vi "ESA-C Objective Transform.vi"(2 "Axis":i32=1 min=1 max=3 step=1, 3 "Is Voltage?":bool, 4 "Input Value":dbl) -> (1 "Output Value":dbl)   [LabVIEW 2010]
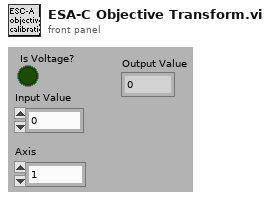
[diagram p1: front panel]
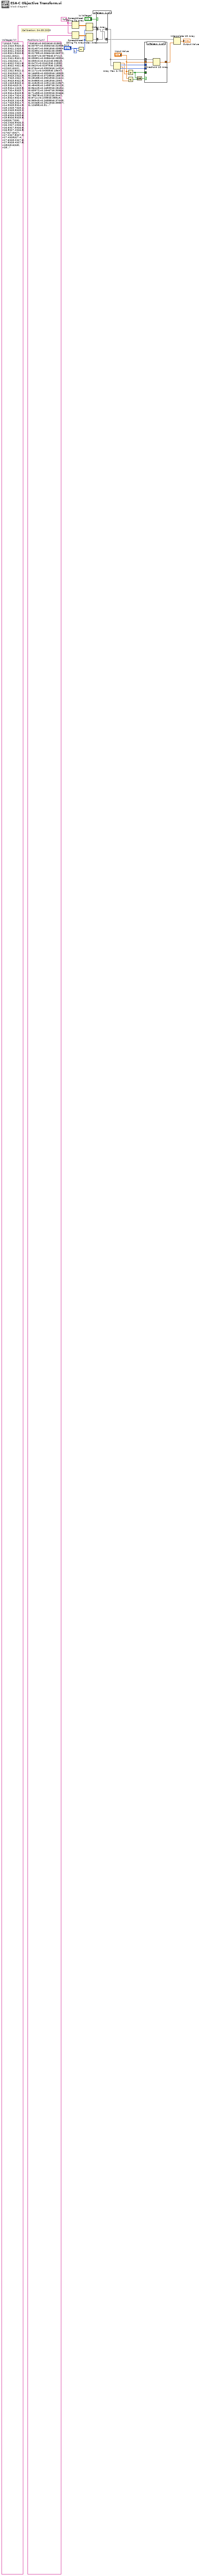
[diagram p0: block diagram]
diagram:
  w2 = "%f" ("Format-String")
  w4 = "0\t0\t0\n0.00206\t0.01582\t0.00797\n0.00364\t0.02598\t0.01407\n0.00618\t0.03864\t0.02391\n0.00461\t0.0389\t0.01785\n0.00664\t0.06372\t0.0257\n0.00796\t0.07414\t0.03081\n0.00864\t0.08594\t0.03344\n0.0122\t0.09613\t0.0472\n0.01613\t0.11592\t0.0624\n0.01975\t0.12826\t0.07644\n0.03026\t0.14314\t0.1171\n0.04305\t0.15647\t0.16659\n0.05309\t0.18503\t0.20543\n0.07285\t0.18573\t0.28188\n0.09015\t0.21641\t0.34883\n0.10815\t0.2394\t0.41849\n0.12511\t0.24567\t0.48409\n0.14587\t0.26123\t0.56443\n0.16533\t0.28494\t0.63972\n0.18467\t0.30966\t0.71458\n0.20333\t0.32666\t0.78678\n0.22512\t0.3447\t0.8711\n0.2495\t0.35813\t0.96543\n0.26998\t0.37045\t1.04468\n0.29125\t0.39557\t1.12698\n0.31199\t0.43186\t1.20721\n0.33041\t0.44995\t1.2785\n0.35642\t0.46128\t1.37913\n0.37679\t0.4852\t1.45795\n0.39894\t0.51012\t1.54367\n0.423\t0.53809\t1.63678\n0.44765\t0.55311\t1.73215\n0.47119\t0.5793\t1.82326\n0.49323\t0.60432\t1.90852\n0.515\t0.63131\t1.99277\n0.54235\t0.65174\t2.0986\n0.56544\t0.67444\t2.18794\n0.59052\t0.70035\t2.28499\n0.61768\t0.72617\t2.39006\n0.64687\t0.74807\t2.50303\n0.67071\t0.77736\t2.59525\n0.69695\t0.79842\t2.69682\n0.72326\t0.82413\t2.79861\n0.75249\t0.851\t2.91173\n0.77818\t0.86434\t3.01111\n0.80787\t0.89958\t3.12601\n0.83626\t0.92291\t3.23587\n0.86609\t0.9444\t3.35128\n0.89348\t0.97648\t3.45728\n0.92459\t1.01656\t3.57766\n0.95407\t1.03769\t3.69172\n0.98644\t1.06928\t3.81698\n1.0145\t1.08591\t3.92557\n1.05304\t1.12184\t4.07469\n1.08169\t1.16283\t4.18554\n1.11425\t1.17713\t4.31154\n1.14477\t1.23843\t4.42962\n1.17871\t1.2712\t4.56095\n1.21176\t1.26837\t4.68883\n1.24316\t1.2797\t4.81034\n1.27406\t1.35775\t4.92992\n1.306\t1.35966\t5.05349\n1.34587\t1.39661\t5.20777\n1.37659\t1.41265\t5.32665\n1.41003\t1.45457\t5.45604\n1.44185\t1.47975\t5.57914\n1.4793\t1.5145\t5.72406\n1.51209\t1.54856\t5.85095\n1.54619\t1.57829\t5.98287\n1.58446\t1.61345\t6.13097\n1.62127\t1.64402\t6.27342\n1.65394\t1.68094\t6.39983\n1.6971\t1.71433\t6.56684\n1.7329\t1.75848\t6.70537\n1.77332\t1.78004\t6.86175\n1.80796\t1.82347\t6.9958\n1.84327\t1.8469\t7.13243\n1.88063\t1.88883\t7.27699\n1.91665\t1.92539\t7.41636\n1.95809\t1.95381\t7.5767\n1.99357\t1.99138\t7.71401\n2.03643\t2.02811\t7.87986\n2.07282\t2.065\t8.02067\n2.11601\t2.10377\t8.18776\n2.15509\t2.14263\t8.33898\n2.19327\t2.17343\t8.48672\n2.23173\t2.20447\t8.63557\n2.27341\t2.23879\t8.79684\n2.31601\t2.27513\t8.96165\n2.35787\t2.31235\t9.12363\n2.39614\t2.3465\t9.27174\n2.44248\t2.40021\t9.45105\n2.4776\t2.44355\t9.58695\n2.52469\t2.44838\t9.76913\n2.56468\t2.51196\t9.92388\n2.60903\t2.54639\t10.0955\n2.65291\t2.5898\t10.2653\n2.69732\t2.63336\t10.43714\n2.73913\t2.65922\t10.59892\n2.78379\t2.70832\t10.77172\n2.82858\t2.74906\t10.94503\n2.86806\t2.77566\t11.0978\n2.91738\t2.8185\t11.28862\n2.96297\t2.8658\t11.46503\n3.00445\t2.90357\t11.62554\n3.05282\t2.95446\t11.81271\n3.09734\t2.98834\t11.98499\n3.14164\t3.02822\t12.1564\n3.18598\t3.06209\t12.32798\n3.2341\t3.1123\t12.51415\n3.27896\t3.14462\t12.68776\n3.32286\t3.18405\t12.8576\n3.37437\t3.23418\t13.05692\n3.41886\t3.27317\t13.22909\n3.4663\t3.32029\t13.41266\n3.51342\t3.34422\t13.59498\n3.55833\t3.39015\t13.76876\n3.61246\t3.42698\t13.97821\n3.6588\t3.47641\t14.15752\n3.70534\t3.51359\t14.33761\n3.75632\t3.57169\t14.53486\n3.80315\t3.59949\t14.71609\n3.85382\t3.64781\t14.91212\n3.89979\t3.69649\t15.09003\n3.94977\t3.73421\t15.28341\n4.00091\t3.77877\t15.4813\n4.04792\t3.82143\t15.6632\n4.09999\t3.87226\t15.86468\n4.14481\t3.918\t16.0381\n4.19552\t3.95085\t16.23433\n4.24804\t4.00483\t16.43755\n4.29611\t4.04561\t16.62355\n4.3445\t4.08787\t16.81079\n4.39609\t4.14791\t17.01041\n4.4472\t4.17144\t17.20818\n4.49829\t4.21375\t17.40587\n4.54788\t4.26894\t17.59774\n4.60011\t4.31296\t17.79985\n4.6533\t4.3514\t18.00569\n4.70481\t4.40255\t18.20499\n4.75815\t4.44984\t18.41138\n4.80998\t4.49487\t18.61196\n4.85901\t4.53422\t18.80166\n4.91528\t4.57675\t19.0194\n4.96618\t4.62801\t19.21633\n5.02209\t4.6768\t19.43268\n5.07231\t4.7086\t19.62702\n5.12469\t4.75743\t19.8297\n5.17561\t4.80586\t20.02672\n5.22927\t4.86141\t20.23436\n5.27506\t4.91224\t20.41152\n5.32744\t4.95287\t20.61423\n5.384\t4.99441\t20.83309\n5.43428\t5.03405\t21.02761\n5.48864\t5.0793\t21.23798\n5.54097\t5.13635\t21.44046\n5.59504\t5.17679\t21.6497\n5.64706\t5.2266\t21.85099\n5.70423\t5.263\t22.07218\n5.75231\t5.30995\t22.25823\n5.80554\t5.35144\t22.46421\n5.85792\t5.4046\t22.66688\n5.91238\t5.44471\t22.87761\n5.9677\t5.49265\t23.09165\n6.02253\t5.53708\t23.30384\n6.07348\t5.58112\t23.50097\n6.12782\t5.63989\t23.71125\n6.17763\t5.6757\t23.90398\n6.23196\t5.71507\t24.11421\n6.2856\t5.76459\t24.32178\n6.33948\t5.81711\t24.53024\n6.39054\t5.84114\t24.72783\n6.44988\t5.87321\t24.95743\n6.50485\t5.94542\t25.17015\n6.55614\t5.99001\t25.36861\n6.60972\t6.03117\t25.57592\n6.66579\t6.07023\t25.79287\n6.71452\t6.1316\t25.98144\n6.76881\t6.1573\t26.19152\n6.82217\t6.24148\t26.39801\n6.87766\t6.24631\t26.61272\n6.93251\t6.29414\t26.82493\n6.98672\t6.34088\t27.03473\n7.04211\t6.39186\t27.24903\n7.09161\t6.42876\t27.44056\n7.14462\t6.48125\t27.64568\n7.20275\t6.52643\t27.87062\n7.2513\t6.56734\t28.0585\n7.30852\t6.61388\t28.27988\n7.36287\t6.65737\t28.49019\n7.41237\t6.71161\t28.68175\n7.46672\t6.7582\t28.89205\n7.52048\t6.764\t29.10006\n7.57284\t6.8349\t29.30268\n7.62522\t6.87743\t29.50533\n7.67605\t6.92471\t29.70205\n7.73309\t6.979\t29.92274\n7.78587\t7.00484\t30.12696\n7.83692\t7.00877\t30.32451\n7.88874\t7.11708\t30.52503\n7.94425\t7.15008\t30.73983\n8.0003\t7.19203\t30.95672\n8.05026\t7.17301\t31.15001\n8.10258\t7.3525\t31.35245\n8.15648\t7.25315\t31.56101\n8.20663\t7.32632\t31.75506\n8.25782\t7.38747\t31.95315\n8.31409\t7.46022\t32.1709\n8.36985\t7.47799\t32.38664\n8.42199\t7.52294\t32.58842\n8.47558\t7.55001\t32.79578\n8.52455\t7.61783\t32.98525\n8.58088\t7.65449\t33.20322\n8.63041\t7.69981\t33.39486\n8.6828\t7.7452\t33.59759\n8.73825\t7.78797\t33.81217\n8.78556\t7.83191\t33.99523\n8.83822\t7.87419\t34.19896\n8.89339\t7.91015\t34.41248\n8.94467\t7.95395\t34.61087\n9.00029\t8.00004\t34.82609\n9.04789\t8.04302\t35.01028\n9.10104\t8.08233\t35.21594\n9.15413\t8.12348\t35.42139\n9.2035\t8.16484\t35.61243\n9.25364\t8.16852\t35.80641\n9.30931\t8.28485\t36.02185\n9.35645\t8.30373\t36.20425\n9.41107\t8.32962\t36.41559\n9.46247\t8.38694\t36.61447\n9.51232\t8.42657\t36.80736\n9.56033\t8.48788\t36.99315\n9.61139\t8.50867\t37.19072\n9.66139\t8.5305\t37.38418\n9.71153\t8.58622\t37.57821\n9.76035\t8.58666\t37.76709\n9.81322\t8.67561\t37.97169\n9.86271\t8.74104\t38.16319\n9.91232\t8.71631\t38.35513\n9.96116\t8.82303\t38.54412\n10.0396\t8.81323\t38.75433\n10.11293\t8.86917\t38.94097\n10.16317\t8.90354\t39.1314\n10.21362\t8.91815\t39.32582\n10.26417\t8.97055\t39.521\n10.31629\t9.0306\t39.7166\n10.36417\t9.09231\t39.91828\n10.4393\t9.09117\t40.10356\n10.51016\t9.13577\t40.30034\n10.56212\t9.19679\t40.48822\n10.6101\t9.23739\t40.66847\n10.65723\t9.27728\t40.86953\n10.70656\t9.31648\t41.05516\n10.75729\t9.32865\t41.23752\n10.80621\t9.38383\t41.4284\n10.85248\t9.42618\t41.62471\n10.90259\t9.44632\t41.814\n10.9494\t9.52148\t41.99304\n10.99657\t9.53135\t42.18693\n11.04455\t9.59795\t42.36807\n11.09076\t9.62348\t42.5506\n11.13748\t9.66961\t42.73625\n11.18797\t9.70076\t42.91506\n11.23827\t9.73559\t43.09583\n11.28985\t9.7884\t43.29121\n11.32964\t9.81555\t43.48582\n11.38187\t9.85709\t43.68541\n11.42597\t9.90824\t43.83939\n11.47253\t9.97563\t44.04148\n11.524\t9.99489\t44.21214\n11.57492\t10.02446\t44.3923\n11.62449\t10.06307\t44.59143\n11.67333\t10.10766\t44.7885\n11.71995\t10.15172\t44.98028\n11.76875\t10.18305\t45.16927\n11.81213\t10.22079\t45.34967\n11.86182\t10.25701\t45.53851\n11.90706\t10.29925\t45.70636\n11.95348\t10.34037\t45.89862\n11.9998\t10.38086\t46.07367\n12.05592\t10.41878\t46.2533\n12.09164\t10.45961\t46.43253\n12.13693\t10.49808\t46.64969\n12.18385\t10.51628\t46.78791\n12.22765\t10.57388\t46.96315\n12.2773\t10.61827\t47.14471\n12.32159\t10.65369\t47.31417\n12.36563\t10.701\t47.50632\n12.41129\t10.72273\t47.67768\n12.45403\t10.78257\t47.84809\n12.49792\t10.81064\t48.02478\n12.54281\t10.85043\t48.19016\n12.58755\t10.88123\t48.35996\n12.63056\t10.93561\t48.53366\n12.67788\t10.95375\t48.70681\n12.7214\t11.00172\t48.87324\n12.76449\t11.0412\t49.05632\n12.80979\t11.07308\t49.22472\n12.85226\t11.11637\t49.39145\n12.90002\t11.16052\t49.56675\n12.93855\t11.19604\t49.73109\n12.98328\t11.23555\t49.9159\n13.03221\t11.26792\t50.06498\n13.07624\t11.30576\t50.23803\n13.1182\t11.35628\t50.42737\n13.16017\t11.38331\t50.59777\n13.21028\t11.42008\t50.76012\n13.25055\t11.46065\t50.9225\n13.2949\t11.49544\t51.11642\n13.33123\t11.54413\t51.27223\n13.37735\t11.5857\t51.44383\n13.418\t11.62174\t51.58444\n13.46358\t11.6533\t51.7629\n13.51193\t11.70144\t51.92018\n13.54756\t11.73269\t52.09654\n13.59149\t11.76663\t52.28364\n13.63076\t11.80746\t52.42152\n13.67299\t11.8394\t52.59147\n13.73724\t11.88143\t52.74344\n13.79991\t11.92458\t52.90683\n13.83781\t11.95047\t53.07778\n13.88384\t11.99286\t53.23312\n13.92377\t12.01943\t53.39796\n13.96633\t12.0551\t53.54462\n14.00794\t12.09251\t53.72271\n14.04791\t12.13338\t53.87721\n14.08947\t12.16338\t54.0419\n14.13105\t12.20913\t54.20292\n14.17595\t12.24683\t54.35758\n14.21676\t12.27849\t54.51839\n14.25537\t12.3022\t54.67927\n14.29735\t12.32687\t54.85302\n14.33217\t12.37302\t55.01095\n14.37497\t12.4095\t55.16035\n14.41315\t12.46333\t55.32275\n14.45041\t12.49714\t55.45752\n14.49464\t12.51998\t55.62312\n14.53416\t12.55584\t55.77086\n14.57249\t12.59911\t55.91502\n14.61628\t12.62685\t56.08619\n14.65589\t12.66232\t56.2391\n14.69349\t12.70316\t56.3874\n14.73356\t12.73113\t56.55685\n14.77638\t12.77004\t56.7101\n14.81337\t12.80714\t56.85563\n14.85036\t12.84273\t57.01066\n14.89207\t12.87774\t57.17633\n14.9287\t12.89924\t57.31949\n14.97201\t12.95137\t57.46261\n15.00902\t12.97001\t57.62402\n15.05224\t13.01897\t57.76575\n15.08843\t13.06468\t57.93331\n15.13144\t13.07355\t58.07655\n15.16988\t13.12448\t58.24376\n15.20703\t13.15448\t58.38381\n15.24318\t13.19253\t58.55022\n15.28321\t13.22758\t58.69896\n15.31889\t13.24679\t58.84272\n15.35389\t13.28935\t58.98259\n15.39295\t13.31942\t59.13749\n15.43233\t13.3592\t59.27555\n15.4735\t13.38902\t59.41097\n15.51074\t13.41598\t59.56213\n15.54896\t13.46041\t59.7145\n15.58342\t13.48785\t59.8738\n15.61957\t13.52485\t60.01793\n15.66229\t13.5602\t60.16579\n15.70146\t13.58365\t60.29914\n15.73583\t13.62554\t60.43902\n15.77056\t13.64647\t60.60433\n15.80613\t13.68735\t60.75589\n15.84725\t13.71912\t60.88887\n15.88168\t13.75632\t61.02328\n15.91807\t13.78847\t61.1609\n15.95758\t13.82242\t61.32002\n15.98736\t13.85868\t61.45323\n16.02927\t13.88936\t61.59407\n16.06444\t13.92294\t61.74695\n16.10392\t13.94828\t61.86215\n16.13877\t13.98304\t62.02434\n16.17486\t14.01765\t62.16043\n16.21007\t14.05858\t62.31319\n16.24608\t14.09598\t62.44802\n16.28212\t14.12115\t62.58768\n16.31712\t14.15602\t62.72394\n16.35364\t14.17255\t62.86328\n16.38596\t14.20573\t63.00273\n16.42832\t14.2371\t63.13815\n16.45836\t14.27324\t63.27945\n16.49525\t14.30763\t63.40452\n16.52868\t14.32702\t63.56843\n16.56779\t14.35572\t63.68466\n16.60098\t14.38991\t63.82743\n16.63625\t14.4269\t63.95679\n16.67306\t14.46493\t64.10811\n16.70432\t14.50426\t64.23654\n16.7403\t14.51645\t64.37301\n16.77452\t14.55184\t64.51543\n16.81095\t14.58351\t64.6364\n16.846\t14.61177\t64.77562\n16.87789\t14.64557\t64.90804\n16.91424\t14.65899\t65.04901\n16.94891\t14.70078\t65.18461\n16.98255\t14.73666\t65.308\n17.01465\t14.77177\t65.44867\n17.05286\t14.79985\t65.58282\n17.08566\t14.82953\t65.71301\n17.12001\t14.86146\t65.8372\n17.15479\t14.88561\t65.98504\n17.19044\t14.92712\t66.11196\n17.22476\t14.95142\t66.24489\n17.25703\t14.98369\t66.37948\n17.28937\t15.00713\t66.51741\n17.32555\t15.05054\t66.6502\n17.35889\t15.08594\t66.77508\n17.39145\t15.12972\t66.90022\n17.42716\t15.17536\t67.04022\n17.45727\t15.18369\t67.16922\n17.49112\t15.22262\t67.29522\n17.52882\t15.26413\t67.43338\n17.56032\t15.28013\t67.5499\n17.59131\t15.31159\t67.68089\n17.62551\t15.33422\t67.82675\n17.65693\t15.3667\t67.94863\n17.68961\t15.40582\t68.06856\n17.72269\t15.42198\t68.2009\n17.75469\t15.46202\t68.32249\n17.78655\t15.49097\t68.44891\n17.81877\t15.51758\t68.57693\n17.85307\t15.55035\t68.70073\n17.88717\t15.56959\t68.82404\n17.91928\t15.60279\t68.9487\n17.95308\t15.63107\t69.0814\n17.98633\t15.65102\t69.21336\n18.01805\t15.68224\t69.3376\n18.05234\t15.70485\t69.46841\n18.08427\t15.73942\t69.59707\n18.11821\t15.75362\t69.7198\n18.15169\t15.78973\t69.85248\n18.18155\t15.81697\t69.97605\n18.21255\t15.84687\t70.10737\n18.24297\t15.87423\t70.23692\n18.27717\t15.90701\t70.35244\n18.30697\t15.93006\t70.47239\n18.34013\t15.96188\t70.59013\n18.36997\t15.99737\t70.72243\n18.40383\t16.01222\t70.83777\n18.43221\t16.04856\t70.96608\n18.46494\t16.06725\t71.08154\n18.49754\t16.09457\t71.21254\n18.52886\t16.12193\t71.32236\n18.56036\t16.15093\t71.44901\n18.59198\t16.17695\t71.57515\n18.61927\t16.21187\t71.69636\n18.649\t16.23614\t71.81826\n18.68104\t16.26521\t71.94059\n18.71093\t16.28839\t72.0462\n18.75639\t16.3168\t72.16122\n18.80228\t16.34569\t72.28522\n18.83393\t16.37416\t72.40085\n18.86222\t16.40412\t72.52265\n18.89461\t16.42178\t72.63089\n18.92701\t16.4535\t72.75432\n18.95818\t16.46829\t72.87682\n18.98897\t16.50818\t72.98629\n19.02153\t16.53456\t73.1116\n19.04958\t16.5552\t73.23696\n19.08469\t16.58307\t73.35759\n19.11312\t16.61305\t73.47673\n19.14191\t16.63315\t73.60273\n19.17381\t16.66148\t73.71124\n19.20398\t16.68534\t73.84711\n19.23484\t16.71109\t73.95711\n19.26137\t16.73776\t74.06852\n19.29306\t16.77008\t74.19195\n19.32035\t16.80204\t74.30869\n19.35077\t16.83371\t74.42811\n19.38289\t16.84493\t74.53077\n19.4094\t16.86013\t74.65336\n19.44052\t16.89874\t74.75896\n19.47154\t16.92062\t74.87668\n19.50039\t16.9547\t75.00096\n19.52605\t16.9683\t75.10354\n19.55592\t17.00169\t75.22399\n19.58496\t17.02601\t75.344\n19.61476\t17.04733\t75.45562\n19.6405\t17.08011\t75.55492\n19.6685\t17.09251\t75.67052\n19.70522\t17.13417\t75.78287\n19.72831\t17.15545\t75.89819\n19.75937\t17.18134\t75.99778\n19.78736\t17.2021\t76.10613\n19.81567\t17.23955\t76.24821\n19.84447\t17.252\t76.33755\n19.87436\t17.27017\t76.45774\n19.90255\t17.30186\t76.56605\n19.93085\t17.33395\t76.67559\n19.9586\t17.36226\t76.78702\n19.98649\t17.37066\t76.90268\n20.01706\t17.41305\t77.01176\n20.04269\t17.42854\t77.12127\n20.07124\t17.46215\t77.22866\n20.10164\t17.4675\t77.33655\n20.12842\t17.49335\t77.45484\n20.15691\t17.54794\t77.55402\n20.18854\t17.55041\t77.6645\n20.21251\t17.58245\t77.78214\n20.2449\t17.59799\t77.88575\n20.25972\t17.64756\t77.99602\n20.29779\t17.65379\t78.1184\n20.32772\t17.67329\t78.21112\n20.35557\t17.70317\t78.33648\n20.3839\t17.71193\t78.3938\n20.41286\t17.76171\t78.54113\n20.44066\t17.76845\t78.65692\n20.46331\t17.80498\t78.76469\n20.50215\t17.8322\t78.8743\n20.52802\t17.84618\t78.98638\n20.55369\t17.87167\t79.09395\n20.5824\t17.89231\t79.18158\n20.60422\t17.91678\t79.33189\n20.63637\t17.95231\t79.432\n20.66195\t17.96685\t79.53131\n20.6868\t17.99216\t79.6424\n20.71605\t18.01686\t79.72685\n20.74309\t18.04313\t79.85123\n20.76869\t18.0887\t79.95023\n20.7967\t18.08542\t80.04637\n20.82399\t18.10391\t80.15957\n20.85074\t18.13152\t80.26418\n20.87875\t18.15564\t80.36325\n20.91072\t18.19027\t80.47164\n20.93438\t18.20115\t80.57722\n20.96502\t18.2259\t80.68075\n20.99354\t18.25154\t80.78913\n21.0176\t18.27389\t80.91281\n21.04038\t18.29835\t81.00439\n21.06843\t18.32377\t81.12294\n21.09194\t18.33802\t81.23329\n21.12167\t18.3649\t81.32638\n21.1461\t18.39318\t81.41452\n21.17404\t18.41672\t81.52307\n21.19846\t18.44837\t81.61405\n21.22317\t18.46084\t81.72907\n21.25075\t18.48664\t81.82362\n21.2759\t18.51315\t81.93173\n21.30247\t18.53912\t82.02623\n21.32951\t18.53823\t82.12184\n21.35711\t18.56413\t82.22856\n21.38057\t18.57543\t82.32585\n21.40892\t18.6245\t82.42868\n21.43286\t18.6425\t82.53331\n21.46008\t18.66423\t82.6401\n21.48643\t18.68286\t82.7309\n21.5093\t18.69689\t82.84057\n21.53548\t18.72749\t82.9332\n21.56315\t18.74745\t83.03855\n21.58571\t18.7758\t83.14049\n21.61576\t18.78836\t83.22898\n21.64147\t18.81738\t83.3303\n21.66509\t18.83643\t83.43738\n21.68878\t18.85858\t83.52466\n21.71493\t18.88702\t83.64093\n21.74174\t18.90549\t83.74042\n21.77049\t18.93402\t83.83181\n21.79525\t18.94273\t83.92348\n21.82169\t18.98017\t84.02467\n21.84886\t18.98979\t84.12842\n21.87395\t19.01421\t84.23963\n21.90038\t19.04852\t84.33546\n21.92375\t19.05596\t84.43778\n21.94827\t19.0921\t84.54288\n21.97373\t19.11039\t84.63997\n21.99848\t19.11082\t84.74225\n22.02571\t19.15572\t84.83269\n22.04885\t19.16836\t84.92755\n22.07378\t19.19153\t85.02609\n22.09591\t19.20787\t85.12184\n22.12003\t19.23069\t85.22722\n22.14532\t19.26051\t85.31674\n22.1699\t19.28207\t85.41323\n22.1979\t19.30049\t85.49884\n22.22431\t19.31385\t85.59216\n22.24921\t19.32734\t85.69002\n22.27301\t19.35886\t85.78514\n22.29907\t19.38431\t85.89349\n22.32422\t19.4096\t85.99567\n22.34873\t19.41513\t86.09204\n22.37409\t19.45116\t86.18414\n22.40103\t19.46861\t86.28497\n22.42534\t19.49256\t86.38227\n22.44761\t19.51241\t86.47713\n22.47616\t19.52943\t86.57524\n22.49892\t19.55184\t86.67948\n22.52259\t19.58113\t86.77356\n22.54693\t19.58976\t86.85972\n22.5746\t19.62248\t86.97018\n22.59786\t19.65009\t87.05828\n22.61926\t19.6512\t87.14985\n22.64467\t19.66778\t87.24405\n22.67039\t19.69852\t87.3511\n22.69452\t19.70844\t87.44111\n22.71639\t19.74781\t87.52393\n22.74274\t19.7596\t87.62224\n22.76791\t19.77999\t87.72176\n22.79197\t19.80082\t87.81515\n22.81893\t19.8349\t87.89977\n22.84029\t19.85228\t88.00173\n22.86512\t19.86181\t88.0991\n22.89062\t19.89347\t88.1922\n22.91421\t19.91645\t88.29653\n22.9374\t19.92765\t88.37917\n22.9627\t19.95425\t88.47525\n22.98885\t19.96448\t88.57393\n23.0103\t19.98953\t88.6652\n23.03169\t20.00388\t88.75493\n23.05774\t20.02385\t88.85282\n23.0806\t20.04697\t88.95404\n23.10336\t20.05217\t89.03704\n23.12726\t20.08926\t89.11979\n23.15075\t20.11042\t89.22059\n23.17304\t20.12387\t89.30905\n23.19804\t20.15183\t89.39712\n23.22063\t20.1657\t89.48959\n23.24326\t20.18455\t89.58051\n23.27001\t20.217\t89.66674\n23.29073\t20.23007\t89.76349\n23.31413\t20.25128\t89.85087\n23.33916\t20.26395\t89.93843\n23.36191\t20.2979\t90.04195\n23.38418\t20.30202\t90.12214\n23.40784\t20.31684\t90.21268\n23.43043\t20.35301\t90.30952\n23.45537\t20.36843\t90.39755\n23.47594\t20.38133\t90.48374\n23.50113\t20.39318\t90.5753\n23.52194\t20.433\t90.66271\n23.54661\t20.44873\t90.75921\n23.56926\t20.47449\t90.8388\n23.59066\t20.48586\t90.93628\n23.61423\t20.50491\t91.01679\n23.6358\t20.51936\t91.11226\n23.65781\t20.53427\t91.1999\n23.68188\t20.57271\t91.2827\n23.70473\t20.58206\t91.37389\n23.72546\t20.59518\t91.45737\n23.74847\t20.62175\t91.54251\n23.77042\t20.63805\t91.63565\n23.79051\t20.66827\t91.72409\n23.8164\t20.67777\t91.80431\n23.84002\t20.68329\t91.89335\n23.85848\t20.71866\t91.97826\n23.87907\t20.72614\t92.05599\n23.90026\t20.74747\t92.15617\n23.92168\t20.77238\t92.24759\n23.94712\t20.78849\t92.31901\n23.96865\t20.81164\t92.39868\n23.98959\t20.82442\t92.48067\n24.01156\t20.85132\t92.56357\n24.03472\t20.85998\t92.66199\n24.05703\t20.86874\t92.7453\n24.07863\t20.90773\t92.82634\n24.10085\t20.90762\t92.91135\n24.12243\t20.94546\t93.00096\n24.1422\t20.95887\t93.0873\n24.16516\t20.96629\t93.17087\n24.18808\t21.00844\t93.25684\n24.20939\t20.99922\t93.34033\n24.23273\t21.0438\t93.41685\n24.25456\t21.05181\t93.50567\n24.27454\t21.07487\t93.59437\n24.29887\t21.09919\t93.67684\n24.31786\t21.11774\t93.76714\n24.34101\t21.13702\t93.85164\n24.36202\t21.15399\t93.92893\n24.38423\t21.17576\t94.02308\n24.40495\t21.19987\t94.09654\n24.4288\t21.2141\t94.18613\n24.44918\t21.23306\t94.26741\n24.47026\t21.25049\t94.35337\n24.49174\t21.27159\t94.43356\n24.51669\t21.29332\t94.52583\n24.53361\t21.30333\t94.6047\n24.55797\t21.33439\t94.68624\n24.57706\t21.34484\t94.76938\n24.60333\t21.38535\t94.8659\n24.62466\t21.3882\t94.93139\n24.64499\t21.41631\t95.02563\n24.6709\t21.42632\t95.09952\n24.6898\t21.44911\t95.20116\n24.71267\t21.46442\t95.28369\n24.73681\t21.49699\t95.36237\n24.75443\t21.5098\t95.46264\n24.77568\t21.53095\t95.53574\n24.79946\t21.55031\t95.62423\n24.81839\t21.56499\t95.71764\n24.8412\t21.60047\t95.78583\n24.86179\t21.61587\t95.86805\n24.88297\t21.62518\t95.96006\n24.90456\t21.64842\t96.03334\n24.9243\t21.67498\t96.1216\n24.94344\t21.68692\t96.20126\n24.96831\t21.69894\t96.28322\n24.98706\t21.72542\t96.36674\n25.00908\t21.74811\t96.44316\n25.03194\t21.76997\t96.5172\n25.052\t21.78833\t96.61345\n25.07531\t21.80278\t96.686\n25.09833\t21.81255\t96.77118\n25.11977\t21.83971\t96.85965\n25.14152\t21.86117\t96.93728\n25.16114\t21.87332\t97.02746\n25.183\t21.89318\t97.11653\n25.20806\t21.91434\t97.1995\n25.22496\t21.93404\t97.28364\n25.24651\t21.93702\t97.35959\n25.27095\t21.95476\t97.44418\n25.29008\t21.96649\t97.54112\n25.31026\t21.98812\t97.60651\n25.32965\t22\t97.68993\n25.35028\t22.01154\t97.7845\n25.37271\t22.03545\t97.85851\n25.39167\t22.05101\t97.9366\n25.41286\t22.07937\t98.01162\n25.43255\t22.07756\t98.09145\n25.45233\t22.0914\t98.17822\n25.47305\t22.11785\t98.2516\n25.49334\t22.13013\t98.33358\n25.51352\t22.15177\t98.40978\n25.53572\t22.16165\t98.48633\n25.55668\t22.18094\t98.5665\n25.57745\t22.19741\t98.64502\n25.59463\t22.21892\t98.72311\n25.61717\t22.22907\t98.809\n25.63704\t22.25629\t98.89011\n25.66001\t22.27915\t98.97045\n25.67658\t22.29864\t99.03696\n25.70101\t22.32365\t99.12415\n25.72204\t22.3418\t99.20104\n25.74392\t22.36304\t99.28991\n25.76369\t22.38093\t99.35402\n25.78399\t22.40089\t99.44858\n25.80408\t22.41687\t99.52993\n25.82308\t22.45056\t99.61463\n25.84352\t22.45513\t99.69111\n\t\t99.76967\n\t\t99.84738\n\t\t99.9209\n\t\t100"  # Positions (µm)
  w3 = "10\t10.7\t10\n10.2\t10.9\t10.2\n10.3\t11.1\t10.3\n10.6\t11.2\t10.6\n10.8\t11.5\t10.8\n11\t11.6\t11\n11.2\t11.8\t11.2\n11.4\t12\t11.4\n11.6\t12.2\t11.6\n11.8\t12.4\t11.8\n12\t12.6\t12\n12.1\t12.8\t12.1\n12.3\t13\t12.3\n12.5\t13.2\t12.5\n12.7\t13.4\t12.7\n12.9\t13.5\t12.9\n13.1\t13.8\t13.1\n13.3\t14\t13.3\n13.5\t14.1\t13.5\n13.7\t14.3\t13.7\n13.9\t14.5\t13.9\n14.1\t14.7\t14.1\n14.3\t14.9\t14.3\n14.5\t15.1\t14.5\n14.7\t15.3\t14.7\n14.9\t15.5\t14.9\n15.1\t15.7\t15.1\n15.2\t15.9\t15.2\n15.4\t16.1\t15.4\n15.6\t16.3\t15.6\n15.8\t16.5\t15.8\n16\t16.7\t16\n16.2\t16.9\t16.2\n16.4\t17.1\t16.4\n16.6\t17.3\t16.6\n16.8\t17.4\t16.8\n17\t17.6\t17\n17.2\t17.8\t17.2\n17.4\t18\t17.4\n17.6\t18.2\t17.6\n17.8\t18.4\t17.8\n18\t18.6\t18\n18.2\t18.8\t18.2\n18.4\t19.1\t18.4\n18.6\t19.2\t18.6\n18.8\t19.4\t18.8\n19\t19.6\t19\n19.1\t19.8\t19.1\n19.4\t20\t19.4\n19.5\t20.2\t19.5\n19.7\t20.3\t19.7\n19.9\t20.6\t19.9\n20.1\t20.7\t20.1\n20.3\t20.9\t20.3\n20.5\t21.1\t20.5\n20.7\t21.4\t20.7\n20.9\t21.6\t20.9\n21.2\t21.7\t21.2\n21.3\t22\t21.3\n21.5\t22.1\t21.5\n21.7\t22.3\t21.7\n21.9\t22.5\t21.9\n22.1\t22.7\t22.1\n22.3\t22.9\t22.3\n22.5\t23.1\t22.5\n22.7\t23.2\t22.7\n22.9\t23.4\t22.9\n23.1\t23.6\t23.1\n23.3\t23.8\t23.3\n23.5\t24\t23.5\n23.7\t24.2\t23.7\n23.9\t24.4\t23.9\n24.1\t24.6\t24.1\n24.3\t24.8\t24.3\n24.5\t25\t24.5\n24.6\t25.2\t24.6\n24.8\t25.4\t24.8\n25.1\t25.6\t25.1\n25.2\t25.8\t25.2\n25.3\t26\t25.3\n25.6\t26.2\t25.6\n25.8\t26.4\t25.8\n26\t26.6\t26\n26.1\t26.8\t26.1\n26.4\t27\t26.4\n26.6\t27.2\t26.6\n26.8\t27.4\t26.8\n27\t27.6\t27\n27.2\t27.8\t27.2\n27.4\t28\t27.4\n27.6\t28.2\t27.6\n27.8\t28.3\t27.8\n28\t28.5\t28\n28.2\t28.7\t28.2\n28.3\t28.9\t28.3\n28.5\t29.1\t28.5\n28.7\t29.3\t28.7\n28.9\t29.5\t28.9\n29.1\t29.7\t29.1\n29.3\t29.9\t29.3\n29.5\t30.1\t29.5\n29.7\t30.2\t29.7\n29.9\t30.5\t29.9\n30.1\t30.7\t30.1\n30.3\t30.9\t30.3\n30.5\t31.1\t30.5\n30.7\t31.3\t30.7\n30.9\t31.4\t30.9\n31.1\t31.6\t31.1\n31.3\t31.8\t31.3\n31.4\t32\t31.4\n31.6\t32.2\t31.6\n31.9\t32.4\t31.9\n32\t32.7\t32\n32.2\t32.8\t32.2\n32.4\t33\t32.4\n32.6\t33.2\t32.6\n32.8\t33.4\t32.8\n33\t33.5\t33\n33.2\t33.8\t33.2\n33.4\t34\t33.4\n33.6\t34.2\t33.6\n33.8\t34.4\t33.8\n34\t34.5\t34\n34.2\t34.7\t34.2\n34.4\t35\t34.4\n34.5\t35.1\t34.5\n34.8\t35.3\t34.8\n34.9\t35.5\t34.9\n35.3\t35.7\t35.3\n35.4\t35.9\t35.4\n35.6\t36.1\t35.6\n35.8\t36.3\t35.8\n35.9\t36.5\t35.9\n36.2\t36.7\t36.2\n36.4\t36.9\t36.4\n36.5\t37.1\t36.5\n36.7\t37.3\t36.7\n36.9\t37.4\t36.9\n37.1\t37.6\t37.1\n37.3\t37.9\t37.3\n37.5\t38.1\t37.5\n37.7\t38.3\t37.7\n37.9\t38.5\t37.9\n38.1\t38.6\t38.1\n38.2\t38.8\t38.2\n38.5\t39\t38.5\n38.7\t39.2\t38.7\n38.9\t39.4\t38.9\n39\t39.6\t39\n39.3\t39.8\t39.3\n39.4\t40\t39.4\n39.6\t40.2\t39.6\n39.8\t40.4\t39.8\n40\t40.5\t40\n40.2\t40.8\t40.2\n40.4\t41\t40.4\n40.6\t41.2\t40.6\n40.8\t41.4\t40.8\n41\t41.6\t41\n41.2\t41.8\t41.2\n41.4\t42\t41.4\n41.6\t42.2\t41.6\n41.8\t42.4\t41.8\n42\t42.5\t42\n42.2\t42.7\t42.2\n42.4\t42.9\t42.4\n42.6\t43.1\t42.6\n42.8\t43.3\t42.8\n43\t43.5\t43\n43.1\t43.7\t43.1\n43.4\t43.9\t43.4\n43.6\t44.1\t43.6\n43.7\t44.3\t43.7\n43.9\t44.4\t43.9\n44.1\t44.6\t44.1\n44.3\t44.9\t44.3\n44.5\t45.1\t44.5\n44.7\t45.3\t44.7\n44.9\t45.5\t44.9\n45.1\t45.6\t45.1\n45.3\t45.8\t45.3\n45.5\t46\t45.5\n45.7\t46.2\t45.7\n45.8\t46.4\t45.8\n46.1\t46.6\t46.1\n46.3\t46.8\t46.3\n46.5\t47\t46.5\n46.7\t47.2\t46.7\n46.9\t47.4\t46.9\n47.1\t47.6\t47.1\n47.3\t47.8\t47.3\n47.5\t48\t47.5\n47.6\t48.2\t47.6\n47.8\t48.4\t47.8\n48\t48.6\t48\n48.2\t48.8\t48.2\n48.4\t49\t48.4\n48.5\t49.2\t48.5\n48.8\t49.3\t48.8\n49\t49.6\t49\n49.2\t49.7\t49.2\n49.4\t50\t49.4\n49.5\t50.2\t49.5\n49.8\t50.3\t49.8\n50\t50.5\t50\n50.2\t50.7\t50.2\n50.4\t50.9\t50.4\n50.6\t51.1\t50.6\n50.8\t51.3\t50.8\n51\t51.5\t51\n51.2\t51.7\t51.2\n51.3\t51.9\t51.3\n51.6\t52.1\t51.6\n51.7\t52.3\t51.7\n51.9\t52.5\t51.9\n52.1\t52.7\t52.1\n52.3\t52.9\t52.3\n52.5\t53.1\t52.5\n52.7\t53.3\t52.7\n52.9\t53.4\t52.9\n53.1\t53.6\t53.1\n53.3\t53.8\t53.3\n53.5\t54\t53.5\n53.7\t54.2\t53.7\n53.9\t54.4\t53.9\n54\t54.6\t54\n54.3\t54.8\t54.3\n54.5\t55\t54.5\n54.7\t55.2\t54.7\n54.9\t55.4\t54.9\n55.1\t55.6\t55.1\n55.3\t55.8\t55.3\n55.5\t56\t55.5\n55.6\t56.2\t55.6\n55.8\t56.4\t55.8\n56\t56.5\t56\n56.2\t56.7\t56.2\n56.4\t56.9\t56.4\n56.6\t57.1\t56.6\n56.8\t57.3\t56.8\n57\t57.5\t57\n57.5\t57.8\t57\n57.6\t57.9\t57.5\n57.8\t58.1\t57.6\n58\t58.3\t57.8\n58.2\t58.5\t58\n58.4\t58.7\t58.2\n58.6\t58.9\t58.4\n59\t59.1\t58.6\n59.2\t59.3\t58.6\n59.4\t59.5\t59\n59.6\t59.7\t59.2\n59.8\t59.9\t59.4\n60\t60.1\t59.6\n60.2\t60.3\t59.8\n60.4\t60.5\t60\n60.6\t60.7\t60.2\n60.7\t60.9\t60.4\n60.9\t61\t60.6\n61.1\t61.3\t60.7\n61.3\t61.5\t60.9\n61.5\t61.7\t61.1\n61.7\t61.8\t61.3\n61.9\t62\t61.5\n62.1\t62.2\t61.7\n62.3\t62.4\t61.9\n62.5\t62.6\t62.1\n62.7\t62.8\t62.3\n62.9\t63\t62.5\n63.1\t63.2\t62.7\n63.3\t63.4\t62.9\n63.5\t63.6\t63.1\n63.7\t63.8\t63.3\n63.9\t64\t63.5\n64.1\t64.2\t63.7\n64.2\t64.4\t63.9\n64.5\t64.6\t64.1\n64.6\t64.7\t64.2\n64.9\t64.9\t64.5\n65.1\t65.2\t64.6\n65.2\t65.3\t64.9\n65.5\t65.6\t65.1\n65.7\t65.7\t65.2\n65.9\t65.9\t65.5\n66.1\t66.1\t65.7\n66.2\t66.4\t65.9\n66.5\t66.5\t66.1\n66.7\t66.7\t66.2\n66.8\t66.9\t66.5\n67\t67.1\t66.7\n67.3\t67.3\t66.8\n67.5\t67.5\t67\n67.7\t67.7\t67.3\n67.8\t67.9\t67.5\n68\t68.1\t67.7\n68.2\t68.3\t67.8\n68.4\t68.5\t68\n68.6\t68.6\t68.2\n68.8\t68.9\t68.4\n69\t69\t68.6\n69.2\t69.3\t68.8\n69.4\t69.5\t69\n69.6\t69.7\t69.2\n69.8\t69.9\t69.4\n70\t70\t69.6\n70.2\t70.2\t69.8\n70.4\t70.4\t70\n70.6\t70.6\t70.2\n70.8\t70.8\t70.4\n70.9\t71\t70.6\n71.2\t71.2\t70.8\n71.3\t71.4\t70.9\n71.6\t71.6\t71.2\n71.7\t71.8\t71.3\n72\t71.9\t71.6\n72.2\t72.2\t71.7\n72.3\t72.4\t72\n72.4\t72.6\t72.2\n72.9\t72.8\t72.3\n73.1\t73\t72.4\n73.4\t73.2\t72.9\n73.5\t73.4\t72.9\n73.7\t73.6\t73.1\n73.9\t73.8\t73.4\n74.1\t74\t73.5\n74.3\t74.2\t73.7\n74.5\t74.4\t73.9\n74.7\t74.6\t74.1\n74.9\t74.7\t74.3\n75.1\t74.9\t74.5\n75.3\t75.1\t74.7\n75.5\t75.3\t74.9\n75.6\t75.5\t75.1\n75.9\t75.7\t75.3\n76\t75.9\t75.5\n76.2\t76.1\t75.6\n76.4\t76.3\t75.9\n76.7\t76.5\t76\n76.9\t76.6\t76.2\n77.1\t76.9\t76.4\n77.3\t77.1\t76.7\n77.5\t77.3\t76.9\n77.7\t77.5\t77.1\n77.8\t77.7\t77.3\n78\t77.9\t77.5\n78.2\t78\t77.7\n78.4\t78.2\t77.8\n78.6\t78.5\t78\n78.8\t78.6\t78.2\n79\t78.8\t78.4\n79.2\t79\t78.6\n79.4\t79.2\t78.8\n79.6\t79.3\t79\n79.9\t79.6\t79.2\n80.1\t79.8\t79.4\n80.2\t80\t79.6\n80.4\t80.2\t79.9\n80.6\t80.4\t80.1\n80.8\t80.7\t80.2\n81\t80.8\t80.4\n81.1\t81\t80.6\n81.4\t81.2\t80.8\n81.6\t81.4\t81\n81.8\t81.6\t81.1\n82\t81.8\t81.4\n82.2\t82\t81.6\n82.4\t82.2\t81.8\n82.6\t82.4\t82\n82.8\t82.6\t82.2\n82.9\t82.8\t82.4\n83.1\t82.9\t82.6\n83.3\t83.1\t82.8\n83.5\t83.3\t82.9\n83.7\t83.5\t83.1\n83.9\t83.8\t83.3\n84.1\t83.9\t83.5\n84.3\t84.1\t83.7\n84.5\t84.4\t83.9\n84.7\t84.6\t84.1\n84.9\t84.7\t84.3\n85.1\t84.9\t84.5\n85.3\t85.1\t84.7\n85.5\t85.3\t84.9\n85.7\t85.5\t85.1\n85.9\t85.7\t85.3\n86.1\t85.9\t85.5\n86.3\t86\t85.7\n86.5\t86.3\t85.9\n86.7\t86.5\t86.1\n86.9\t86.6\t86.3\n87.1\t86.9\t86.5\n87.3\t87.1\t86.7\n87.5\t87.2\t86.9\n87.7\t87.5\t87.1\n87.9\t87.7\t87.3\n88\t87.8\t87.5\n88.2\t88\t87.7\n88.4\t88.2\t87.9\n88.6\t88.4\t88\n88.8\t88.6\t88.2\n89.1\t88.8\t88.4\n89.2\t89\t88.6\n89.4\t89.2\t88.8\n89.6\t89.4\t89.1\n89.8\t89.6\t89.2\n90\t89.8\t89.4\n90.2\t90\t89.6\n90.4\t90.2\t89.8\n90.6\t90.4\t90\n90.8\t90.6\t90.2\n91\t90.8\t90.4\n91.1\t91\t90.6\n91.4\t91.2\t90.8\n91.6\t91.4\t91\n91.8\t91.7\t91.1\n92\t92\t91.4\n92.1\t92.1\t91.6\n92.4\t92.3\t91.8\n92.6\t92.6\t92\n92.8\t92.8\t92.1\n93\t93\t92.4\n93.1\t93.1\t92.6\n93.4\t93.3\t92.8\n93.5\t93.5\t93\n93.7\t93.7\t93.1\n93.9\t93.9\t93.4\n94.1\t94.1\t93.5\n94.3\t94.3\t93.7\n94.5\t94.6\t93.9\n94.7\t94.7\t94.1\n95\t94.9\t94.3\n95.1\t95.1\t94.5\n95.3\t95.3\t94.7\n95.5\t95.5\t95\n95.6\t95.7\t95.1\n95.9\t95.9\t95.3\n96.1\t96\t95.5\n96.3\t96.3\t95.6\n96.5\t96.4\t95.9\n96.7\t96.6\t96.1\n96.9\t96.8\t96.3\n97.1\t97\t96.5\n97.3\t97.2\t96.7\n97.5\t97.4\t96.9\n97.8\t97.6\t97.1\n97.9\t97.8\t97.3\n98.1\t98\t97.5\n98.2\t98.2\t97.8\n98.5\t98.4\t97.9\n98.7\t98.6\t98.1\n98.9\t98.8\t98.2\n99.1\t99\t98.5\n99.3\t99.2\t98.7\n99.5\t99.4\t98.9\n99.7\t99.6\t99.1\n99.8\t99.8\t99.3\n100.1\t100\t99.5\n100.4\t100.2\t99.7\n100.6\t100.4\t99.8\n100.8\t100.6\t100.1\n101\t100.8\t100.4\n101.2\t101\t100.4\n101.4\t101.1\t100.6\n101.7\t101.3\t100.8\n101.8\t101.5\t101\n102\t101.7\t101.2\n102.2\t102\t101.4\n102.4\t102.1\t101.7\n102.6\t102.3\t101.8\n102.8\t102.5\t102\n103\t102.7\t102.2\n103.2\t102.9\t102.4\n103.4\t103.1\t102.6\n103.6\t103.3\t102.8\n103.8\t103.5\t103\n104\t103.7\t103.2\n104.2\t103.9\t103.4\n104.4\t104.1\t103.6\n104.6\t104.3\t103.8\n104.8\t104.5\t104\n105\t104.7\t104.2\n105.2\t104.9\t104.4\n105.3\t105.1\t104.6\n105.5\t105.3\t104.8\n105.7\t105.5\t105\n106\t105.7\t105.2\n106.2\t105.9\t105.3\n106.3\t106.1\t105.5\n106.6\t106.3\t105.7\n106.8\t106.5\t106\n107\t106.7\t106.2\n107.2\t106.8\t106.3\n107.3\t107\t106.6\n107.5\t107.2\t106.8\n107.8\t107.4\t107\n108\t107.6\t107.2\n108.1\t107.8\t107.3\n108.4\t108\t107.5\n108.5\t108.2\t107.8\n108.7\t108.4\t108\n108.9\t108.7\t108.1\n109.2\t108.8\t108.4\n109.3\t109\t108.5\n109.5\t109.2\t108.7\n109.7\t109.4\t108.9\n109.9\t109.6\t109.2\n110.1\t109.8\t109.3\n110.3\t110\t109.5\n110.5\t110.1\t109.7\n110.7\t110.4\t109.9\n110.9\t110.6\t110.1\n111.1\t110.8\t110.3\n111.3\t111\t110.5\n111.5\t111.2\t110.7\n111.7\t111.3\t110.9\n111.9\t111.5\t111.1\n112.1\t111.7\t111.3\n112.3\t111.9\t111.5\n112.5\t112.1\t111.7\n112.7\t112.3\t111.9\n112.9\t112.4\t112.1\n113.1\t112.7\t112.3\n113.3\t112.9\t112.5\n113.5\t113.1\t112.7\n113.7\t113.3\t112.9\n113.9\t113.5\t113.1\n114.1\t113.7\t113.3\n114.3\t113.9\t113.5\n114.4\t114.1\t113.7\n114.6\t114.3\t113.9\n114.8\t114.5\t114.1\n115\t114.7\t114.3\n115.2\t114.9\t114.4\n115.4\t115.1\t114.6\n115.6\t115.3\t114.8\n115.7\t115.5\t115\n116\t115.7\t115.2\n116.2\t115.9\t115.4\n116.4\t116.1\t115.6\n116.6\t116.2\t115.7\n116.8\t116.4\t116\n117\t116.6\t116.2\n117.2\t116.8\t116.4\n117.4\t117\t116.6\n117.6\t117.2\t116.8\n117.8\t117.4\t117\n118\t117.6\t117.2\n118.2\t117.8\t117.4\n118.4\t118\t117.6\n118.6\t118.2\t117.8\n118.8\t118.4\t118\n119\t118.6\t118.2\n119.2\t118.8\t118.4\n119.3\t119\t118.6\n119.6\t119.2\t118.8\n119.7\t119.3\t119\n119.9\t119.6\t119.2\n120.1\t119.7\t119.3\n120.4\t120\t119.6\n120.6\t120.1\t119.7\n120.7\t120.4\t119.9\n121\t120.5\t120.1\n121.2\t120.7\t120.4\n121.4\t120.9\t120.6\n121.5\t121.1\t120.7\n121.7\t121.3\t121\n121.9\t121.5\t121.2\n122.1\t121.7\t121.4\n122.3\t121.9\t121.5\n122.5\t122.1\t121.7\n122.7\t122.3\t121.9\n122.9\t122.5\t122.1\n123.1\t122.7\t122.3\n123.3\t122.9\t122.5\n123.5\t123.1\t122.7\n123.7\t123.3\t122.9\n123.9\t123.5\t123.1\n124\t123.7\t123.3\n124.3\t123.9\t123.5\n124.5\t124.1\t123.7\n124.7\t124.3\t123.9\n124.9\t124.5\t124\n125.1\t124.6\t124.3\n125.3\t124.9\t124.5\n125.5\t125.1\t124.7\n125.7\t125.3\t124.9\n125.9\t125.5\t125.1\n126.1\t125.6\t125.3\n126.3\t125.9\t125.5\n126.4\t126.1\t125.7\n126.6\t126.3\t125.9\n126.8\t126.4\t126.1\n127\t126.7\t126.3\n127.2\t126.8\t126.4\n127.4\t127\t126.6\n127.6\t127.2\t126.8\n127.8\t127.4\t127\n128.1\t127.6\t127.2\n128.2\t127.8\t127.4\n128.4\t128\t127.6\n128.6\t128.2\t127.8\n128.8\t128.4\t128.1\n129\t128.5\t128.2\n129.2\t128.8\t128.4\n129.4\t129\t128.6\n129.6\t129.2\t128.8\n129.8\t129.3\t129\n130\t129.6\t129.2\n130.2\t129.7\t129.4\n130.4\t129.9\t129.6\n130.6\t130.1\t129.8\n130.8\t130.3\t130\n131\t130.5\t130.2\n131.2\t130.8\t130.4\n131.4\t130.9\t130.6\n131.5\t131.1\t130.8\n131.7\t131.3\t131\n132\t131.5\t131.2\n132.2\t131.6\t131.4\n132.3\t131.9\t131.5\n132.5\t132.1\t131.7\n132.7\t132.3\t132\n132.9\t132.5\t132.2\n133.1\t132.7\t132.3\n133.3\t132.9\t132.5\n133.5\t133.1\t132.7\n133.7\t133.3\t132.9\n133.9\t133.5\t133.1\n134.1\t133.7\t133.3\n134.3\t133.9\t133.5\n134.5\t134.1\t133.7\n134.7\t134.2\t133.9\n134.9\t134.5\t134.1\n135.1\t134.6\t134.3\n135.3\t134.8\t134.5\n135.5\t135\t134.7\n135.7\t135.2\t134.9\n135.9\t135.4\t135.1\n136.1\t135.6\t135.3\n136.3\t135.8\t135.5\n136.5\t135.9\t135.7\n136.7\t136.2\t135.9\n136.9\t136.4\t136.1\n137\t136.6\t136.3\n137.3\t136.8\t136.5\n137.5\t137\t136.7\n137.7\t137.2\t136.9\n137.8\t137.4\t137\n138\t137.6\t137.3\n138.3\t137.8\t137.5\n138.5\t138\t137.7\n138.6\t138.2\t137.8\n138.8\t138.4\t138\n139\t138.6\t138.3\n139.2\t138.7\t138.5\n139.4\t138.9\t138.6\n139.6\t139.1\t138.8\n139.8\t139.3\t139\n140\t139.5\t139.2\n140.2\t139.7\t139.4\n140.4\t139.9\t139.6\n140.6\t140.1\t139.8\n140.8\t140.3\t140\n141\t140.5\t140.2\n141.2\t140.7\t140.4\n141.4\t140.9\t140.6\n141.6\t141.1\t140.8\n141.8\t141.3\t141\n141.9\t141.5\t141.2\n142.2\t141.7\t141.4\n142.4\t141.9\t141.6\n142.5\t142\t141.8\n142.8\t142.3\t141.9\n143\t142.5\t142.2\n143.2\t142.6\t142.4\n143.4\t142.8\t142.5\n143.6\t143\t142.8\n143.7\t143.2\t143\n143.9\t143.4\t143.2\n144.1\t143.6\t143.4\n144.3\t143.8\t143.6\n144.5\t144\t143.7\n144.7\t144.2\t143.9\n144.9\t144.5\t144.1\n145.1\t144.6\t144.3\n145.3\t144.8\t144.5\n145.5\t145\t144.7\n145.7\t145.2\t144.9\n145.8\t145.4\t145.1\n146.1\t145.6\t145.3\n146.3\t145.8\t145.5\n146.5\t146\t145.7\n146.7\t146.2\t145.8\n146.9\t146.4\t146.1\n147.1\t146.6\t146.3\n147.3\t146.8\t146.5\n147.5\t147\t146.7\n147.7\t147.2\t146.9\n147.9\t147.4\t147.1\n148.1\t147.6\t147.3\n148.3\t147.7\t147.5\n148.5\t147.9\t147.7\n148.7\t148.1\t147.9\n148.8\t148.3\t148.1\n149\t148.5\t148.3\n149.2\t148.7\t148.5\n149.4\t148.9\t148.7\n149.6\t149.1\t148.8\n149.9\t149.3\t149\n150.1\t149.5\t149.2\n150.3\t149.7\t149.4\n150.5\t149.9\t149.6\n150.6\t150.1\t149.9\n150.8\t150.3\t150.1\n151\t150.5\t150.3\n151.2\t150.7\t150.5\n151.4\t150.8\t150.6\n151.6\t151\t150.8\n151.8\t151.2\t151\n152\t151.4\t151.2\n152.2\t151.6\t151.4\n152.4\t151.8\t151.6\n152.6\t152\t151.8\n152.8\t152.2\t152\n153\t152.4\t152.2\n153.2\t152.6\t152.4\n153.4\t152.8\t152.6\n153.6\t153\t152.8\n153.8\t153.2\t153\n154\t153.4\t153.2\n154.2\t153.6\t153.4\n154.4\t153.8\t153.6\n154.6\t154\t153.8\n154.8\t154.2\t154\n155\t154.4\t154.2\n155.2\t154.6\t154.4\n155.4\t154.8\t154.6\n155.6\t155\t154.8\n155.8\t155.2\t155\n155.9\t155.4\t155.2\n156.1\t155.6\t155.4\n156.3\t155.8\t155.6\n156.5\t155.9\t155.8\n156.7\t156.1\t155.9\n156.9\t156.3\t156.1\n\t\t156.3\n\t\t156.5\n\t\t156.7\n\t\t156.9"  # Voltages (V)
  # "Calibration: 04.05.2020"
  n1 = Spreadsheet String To Array(format string=w2, spreadsheet string=w3) -> (array=w6:dbl[][])  [unwired: 2 in]
  n2 = Spreadsheet String To Array(format string=w2, spreadsheet string=w4) -> (array=w5:dbl[][])  [unwired: 2 in]
  n3 = Subtract(x="Axis", y=1) -> (x-y=w1:i32)
  n4 = Index Array(array=w6, index (col)=w1) -> (element=w10:dbl[])  [unwired: 1 in]
  n5 = Index Array(array=w5, index (col)=w1) -> (element=w11:dbl[])  [unwired: 1 in]
  n6 = case shown="False" "Is Voltage?" {
    tunnel: [w24 w27] -> w22
    tunnel: w10 -> [w25 w27]
    tunnel: [w25 w26] -> w12
    tunnel: w11 -> [w24 w26]
    frame False {
    }
    frame True {
    }
  }
  n7 = Array Max & Min(array=w22) -> (max value=w15:dbl, max index (indices)=w19:i32, min value=w16:dbl, min index (indices)=w20:i32)
  n8 = Greater?(x="Input Value", y=w15) -> (0:w18:bool)
  n9 = Less?(x="Input Value", y=w16) -> (x < y?=w14:bool)
  n10 = Or(x=w18, y=w14) -> (x .or. y?=w17:bool)
  n11 = case shown="False" w17 {
    tunnel: w18 -> [_ w34]
    tunnel: [w28 w33] -> w21
    tunnel: w19 -> [_ w32]
    tunnel: w20 -> [_ w31]
    tunnel: w22 -> [w30 _]
    tunnel: "Input Value" -> [w29 _]
    frame False {
      n12 = Threshold 1D Array(2:w29, 3:w30) -> (0:w28:dbl)  [unwired: 1 in]
    }
    frame True {
      n13 = case shown="True" w34 {
        tunnel: [w35 w36] -> w33
        tunnel: w32 -> [_ w36]
        tunnel: w31 -> [w35 _]
        frame False {
        }
        frame True {
        }
      }
    }
  }
  n14 = Interpolate 1D Array(1:w21, 2:w12) -> (0:→"Output Value":dbl)
